vi "Try Read Message.vi"(8 "error in (no error)":errorcluster, 9 "timeout ms (100)":i32=100, 11 "OBS in":refnum<class "OBS.lvclass">) -> (0 "error out":errorcluster, 1 "Timeout":bool, 2 "Data":string, 3 "OBS out":refnum<class "OBS.lvclass">)   [LabVIEW 2020, in "obs-websocket.lvlib" / "OBS.lvclass"]
uses:
  OBS.lvclass
  OBS.lvclass/OBS.ctl
  <vilib>/MediaMongrels Ltd/WebSockets/WebSockets/WebSocket Client/WebSocket Client.lvclass
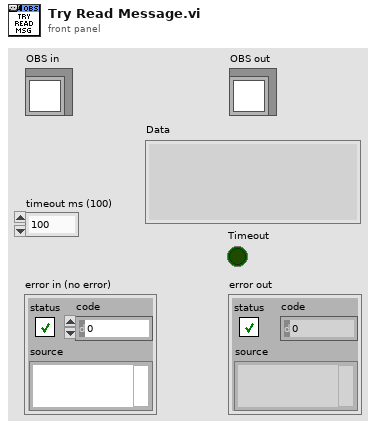
[diagram p1: front panel]
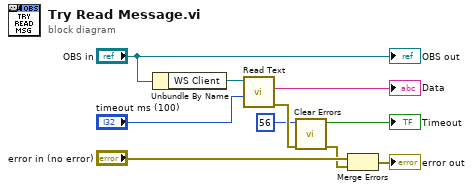
[diagram p0: block diagram]
diagram:
  n1 = Unbundle By Name("OBS in") -> ("WS Client"=w8:refnum<class "WebSocket Client.lvclass">)
  n2 = call-dynamic "Read Text.vi"("timeout ms (5000)"="timeout ms (100)", "WebSocket in"=w8) -> ("error out"=w6:errorcluster, "Data"=→"Data":string)  [unwired: 7 in, 1 out]
  n3 = call <vilib>:"Clear Errors.vi"("error in (no error)"=w6, "specific error code to clear (0: all)"=56) -> ("error out"=w1:errorcluster, "specific error cleared?"=→"Timeout":bool)  [unwired: 4 in]
  n4 = Merge Errors("error in (no error)", w1) -> (→"error out":errorcluster)
  "OBS out" <- "OBS in"
